vi "Update.vi"(8 "error in (no error)":errorcluster, 10 "Message in":refnum<class "UpdateMessage.lvclass">, 11 "ServiceManager in":refnum<class "ServiceManager.lvclass">) -> (0 "error out":errorcluster, 3 "ServiceManager out":refnum<class "ServiceManager.lvclass">)   [LabVIEW 2012, in "ServiceManager.lvclass"]
doc: "The update method processes the command 'update'. \n\nThe command 'update' is used for receiving new values to be set to the private data of the class. This could be seen as a public set method for setting new parameters to the private class data."
uses:
  ServiceManager.lvclass
  Murmex/LabVIEW/Murmex/UpdateMessage/UpdateMessage.lvclass
  Murmex/LabVIEW/Murmex/Murmex/Murmex.lvclass
panel:
  # "This method is called when the UPDATE\ntrigger is sent. \n\nOverride this method when your component needs to\nrespond to this trigger. \n\nCall parent for proper implementation"
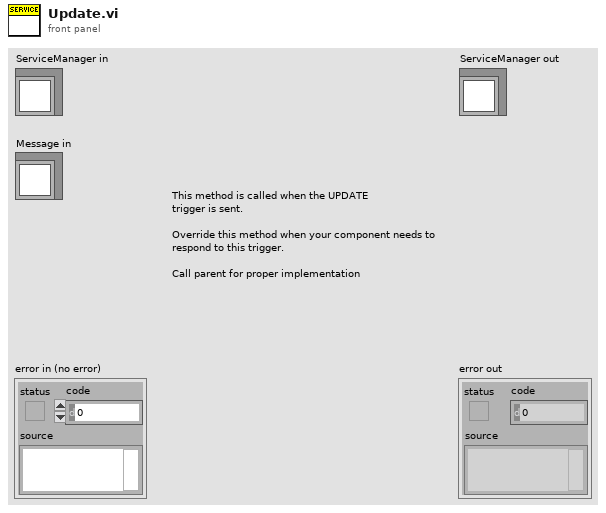
[diagram p1: front panel]
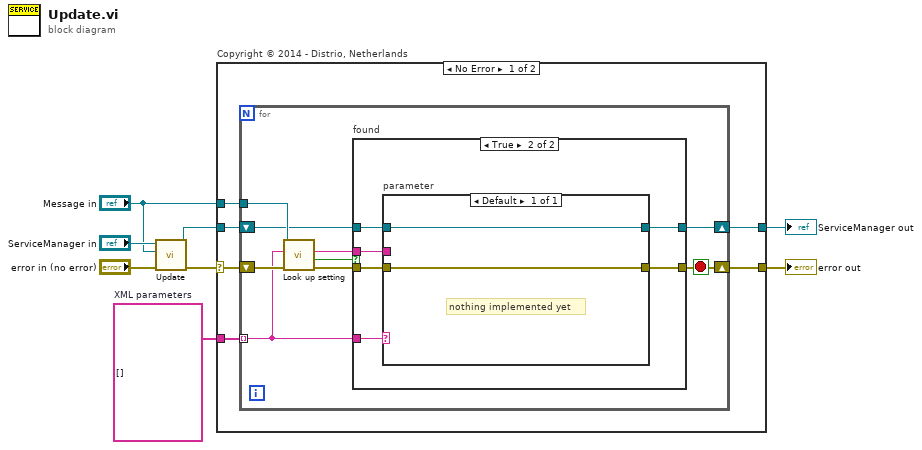
[diagram p0: block diagram]
diagram:
  w4 = string[] []  # XML parameters
  n1 = call-parent "Update.vi"("error in (no error)"="error in (no error)", "Message in"="Message in", "Murmex in"="ServiceManager in") -> ("error out"=w6:errorcluster, "Murmex out"=w5:refnum<class "ServiceManager.lvclass">)  [unwired: 7 in]
  n2 = case "Copyright © 2014 - Distrio, Netherlands" shown="No Error" w6 {
    selector: w6 -> [w14 w34]
    tunnel: w5 -> [w11 w35]
    tunnel: w4 -> [w12 _]
    tunnel: "Message in" -> [w13 _]
    tunnel: [w10 w34] -> w3
    tunnel: [w9 w35] -> w2
    frame No Error {
      n3 = for {
        tunnel: w13 -> [w22]
        tunnel: w12 -> [w19] mode=indexing
        shift-right: [w15] -> w10
        shift-left: w14 -> [w23]
        shift-right: [w16] -> w9
        shift-left: w11 -> [w17]
        stop <- w15 stop-if-true
        n4 = call "Look up setting.vi"("error in (no error)"=w23, "tag name"=w19, "UpdateMessage in"=w22) -> ("error out"=w18:errorcluster, "found?"=w21:bool, "value"=w20:string)  [unwired: 5 in, 1 out]
        n5 = case "found" shown="True" w21 {
          tunnel: w20 -> [_ w28]
          tunnel: w19 -> [_ w31]
          tunnel: w18 -> [w24 w30]
          tunnel: w17 -> [w25 w29]
          tunnel: [w24 w27] -> w15
          tunnel: [w25 w26] -> w16
          frame False {
          }
          frame True {
            n6 = case "parameter" shown="Default" w31 {
              tunnel: w30 -> [w32]
              tunnel: w29 -> [w33]
              tunnel: w28 -> [_]
              tunnel: [w32] -> w27
              tunnel: [w33] -> w26
              frame Default {
                # "nothing implemented yet"
              }
            }
          }
        }
      }
    }
    frame Error {
    }
  }
  "error out" <- w3
  "ServiceManager out" <- w2
